vi "(SubVI) Calc. Smith-eFJC extension.vi"(0 "ssDNA Length (nt)":dbl, 1 "nm/nt":dbl=0.56, 2 "Force (pN)":dbl, 3 "Persistence length (nm)":dbl=0.75, 4 "Elastic modulus (pN)":dbl=800.0) -> (6 "Extension (nm)":dbl)   [LabVIEW 2014]
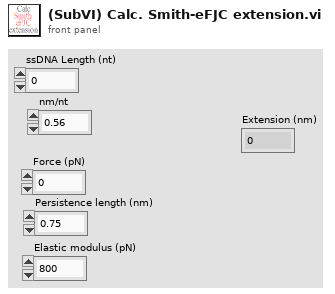
[diagram p1: front panel]
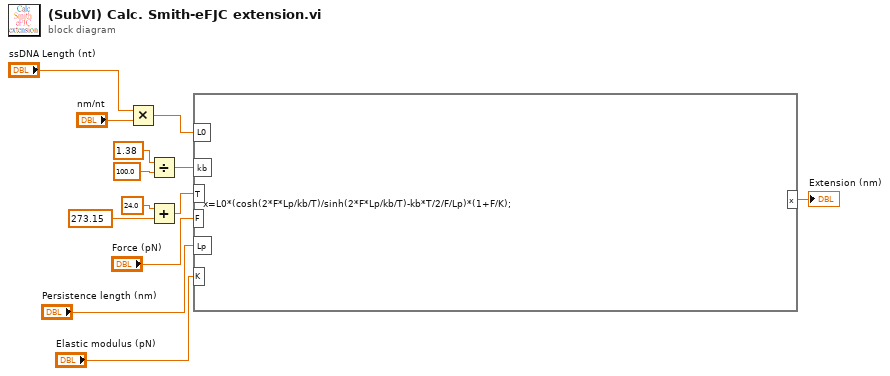
[diagram p0: block diagram]
diagram:
  n1 = Multiply(x="ssDNA Length (nt)", y="nm/nt") -> (x*y=w12:dbl)
  n2 = Divide(x=1.38 ("input variable"), y=100.0) -> (x/y=w9:dbl)
  n3 = Add(x=24.0 ("input variable"), y=273.15) -> (x+y=w6:dbl)
  n4 = formula code="x=L0*(cosh(2*F*Lp/kb/T)/sinh(2*F*Lp/kb/T)-kb*T/2/F/Lp)*(1+F/K);"("L0"=w12, "kb"=w9, "T"=w6, "F"="Force (pN)", "Lp"="Persistence length (nm)", "K"="Elastic modulus (pN)") -> ("x"=→"Extension (nm)":dbl)
